vi "nominal asset attach dataset commit.vi"(7 "out_asset":i32, 8 "error in (no error)":errorcluster, 9 "staging":i32, 10 "rid":string, 11 "client":i32) -> (0 "error out":errorcluster, 3 "function return":i32, 5 "out_asset out":i32)   [LabVIEW 2020, in "client.lvlib"]
doc: "int32_t nominal_asset_attach_dataset_commit(int32_t client,\n const char *rid,\n int32_t staging,\n int32_t *out_asset);"
uses:
  client.lvlib
  bin/nominalClient_64.dll
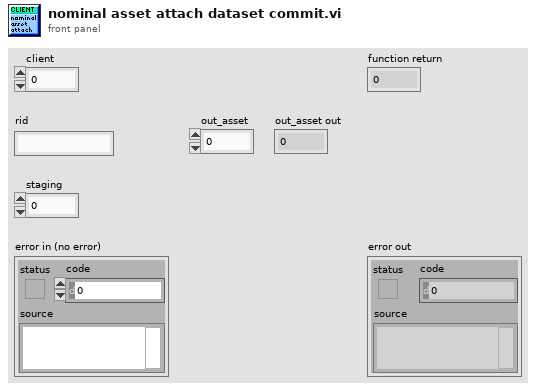
[diagram p1: front panel]
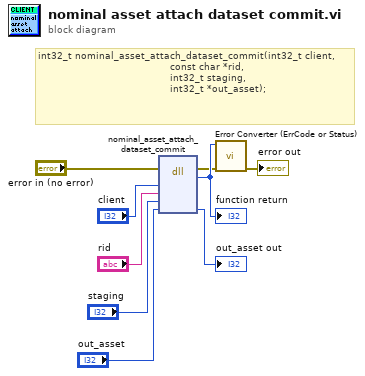
[diagram p0: block diagram]
diagram:
  # "int32_t nominal_asset_attach_dataset_commit(int32_t client,\n                                            const char *rid,\n                                            int32_t staging,\n                                            int32_t *out_asset);"
  n1 = dll-call lib="C:/code/labview-client-rs/lv_src/bin/nominalClient_*.*" fn="nominal_asset_attach_dataset_commit"(error in="error in (no error)", "client"="client", "rid"="rid", "staging"="staging", "out_asset"="out_asset") -> (error out=w2:errorcluster, w9:i32, "out_asset"=→"out_asset out":i32)  [unwired: 5 in, 1 out]
  "function return" <- w9
  n2 = call "Error Converter (ErrCode or Status).vi"("error in (no error)"=w2, "error code"=w9) -> ("error out"=→"error out":errorcluster)  [unwired: 9 in]
